vi "Periodic Tasks.vi"(8 "error in":errorcluster) -> ()   [LabVIEW 2023]
doc: "This VI runs in parallel to other robot code. It can contain as many user-defined periodic loops as you need. These can carry out PID or other sorts of timed response."
uses:
  MHZLib/Variables and Definitions/DB Auton Data.ctl
  <vilib>/Rock Robotics/WPI/ThirdParty/REV Robotics/REVLib/Typedef/Spark MAX Control Type.ctl
  <vilib>/Analysis/coordinate.llb/Angle Range (Degree).ctl
  <vilib>/Analysis/coordinate.llb/Angle Units.ctl
  MHZLib/Variables and Definitions/Auto_Values.ctl
  <vilib>/Rock Robotics/WPI/ThirdParty/Phoenix-LabVIEW/Pigeon IMU/CTRE_PigeonIMU_TareType.ctl
  c1e43d3c-3167-4efa-a61c-2a6e94be98fe.vi
  fdb43fbb-35d8-47d4-8d64-3b5a3af586d8.vi
  8a72de37-8128-41b9-abfb-9e0f917d53f3.vi
  <vilib>/Analysis/coordinate.llb/Wrap Angle (array).vi
  MHZLib/Variables and Definitions/Robot Global Data.vi
  <vilib>/Rock Robotics/Network Tables/NT Read Boolean.vi
  <vilib>/Rock Robotics/Network Tables/NT Read Float.vi
  <vilib>/addons/control/pid/pid.llb/PID (DBL).vi
  <vilib>/Rock Robotics/Network Tables/NT Write Number.vi
  <vilib>/Analysis/coordinate.llb/Angle Rotation (array).vi
  <vilib>/Analysis/coordinate.llb/Wrap Angle (scalar).vi
  <vilib>/Rock Robotics/WPI/ThirdParty/Phoenix-LabVIEW/Pigeon IMU/CTRE_PigeonIMU_GetYPR.vi
  <vilib>/Analysis/coordinate.llb/2D Cartesian Coordinate Rotation (Scalar).vi
  <vilib>/Rock Robotics/Network Tables/NT Read Numeric Array.vi
  <vilib>/Analysis/NI_AAL_Angle.lvlib
  <vilib>/Analysis/NI_AALPro.lvlib
  <vilib>/addons/control/pid/NI_PID_pid.lvlib
panel:
  in  "Speaker Pos":dbl
  in  "Amp Pos":dbl
  in  "Travel Pos":dbl
  in  "Intake Buffer":i16
  in  "Deliver Throttle":dbl
  in  "Intake Throttle":dbl
  out "Current Location":T1 {"Shooter Throttle" min=-360.0 max=360.0}
  in  "Strafe Tolerance":dbl
  in  "Rotate Tolerance":dbl
  in  "Target Rot":dbl
  in  "Target Y":dbl
  in  "Target X":dbl
  in  "Cancel":bool
  in  "Go To":bool
  in  "PID x":T2={"proportional gain (Kc)"=1.0, "integral time (Ti, min)"=0.01, "derivative time (Td, min)"=0.0} {"derivative time (Td, min)" format="%.3f"; "integral time (Ti, min)" format="%.3f"; "proportional gain (Kc)" format="%.3f"}
  in  "PID y":T2={"proportional gain (Kc)"=1.0, "integral time (Ti, min)"=0.01, "derivative time (Td, min)"=0.0} {"derivative time (Td, min)" format="%.3f"; "integral time (Ti, min)" format="%.3f"; "proportional gain (Kc)" format="%.3f"}
  in  "PID rot":T2={"proportional gain (Kc)"=1.0, "integral time (Ti, min)"=0.01, "derivative time (Td, min)"=0.0} {"derivative time (Td, min)" format="%.3f"; "integral time (Ti, min)" format="%.3f"; "proportional gain (Kc)" format="%.3f"}
  in  "Pod Offset":dbl[](array[numeric])=[90.0, 180.0, -90.0, 0.0]
  in  "Drive Mode":bool=TRUE caption="Gyro"
  in  "Reinit Gyro":bool
  out "BR Position":dbl
  out "FR Position":dbl
  out "BL Position":dbl
  out "FL Position":dbl
  out "Right X":dbl
  out "Left Y":dbl
  out "Left X":dbl
  in  "Drive Throttle":dbl
  in  "Drive dband":dbl
  in  "Steer dband":dbl
  out "FL Drive":dbl
  out "BL Drive":dbl
  out "FR Drive":dbl
  out "BR Drive":dbl
  out "Yaw":dbl
  in  "BR Steer":dbl
  in  "FR Steer":dbl
  in  "BL Steer":dbl
  in  "FL Steer":dbl
  # "I should probably look into why attempting to remove\nthis \"error in\" var completely breaks PT... or better yet,\nI should learn to implement proper error handling."
  # "This is some manual setpoint stuff for testing purposes"
  # "FL\n\nFR\n\nBR\n\nBL"
  # "ALWAYS have a backup plan!"
  # "Takes precedence\nfrom Tol"
  # "Relative"
  # "Absolute"
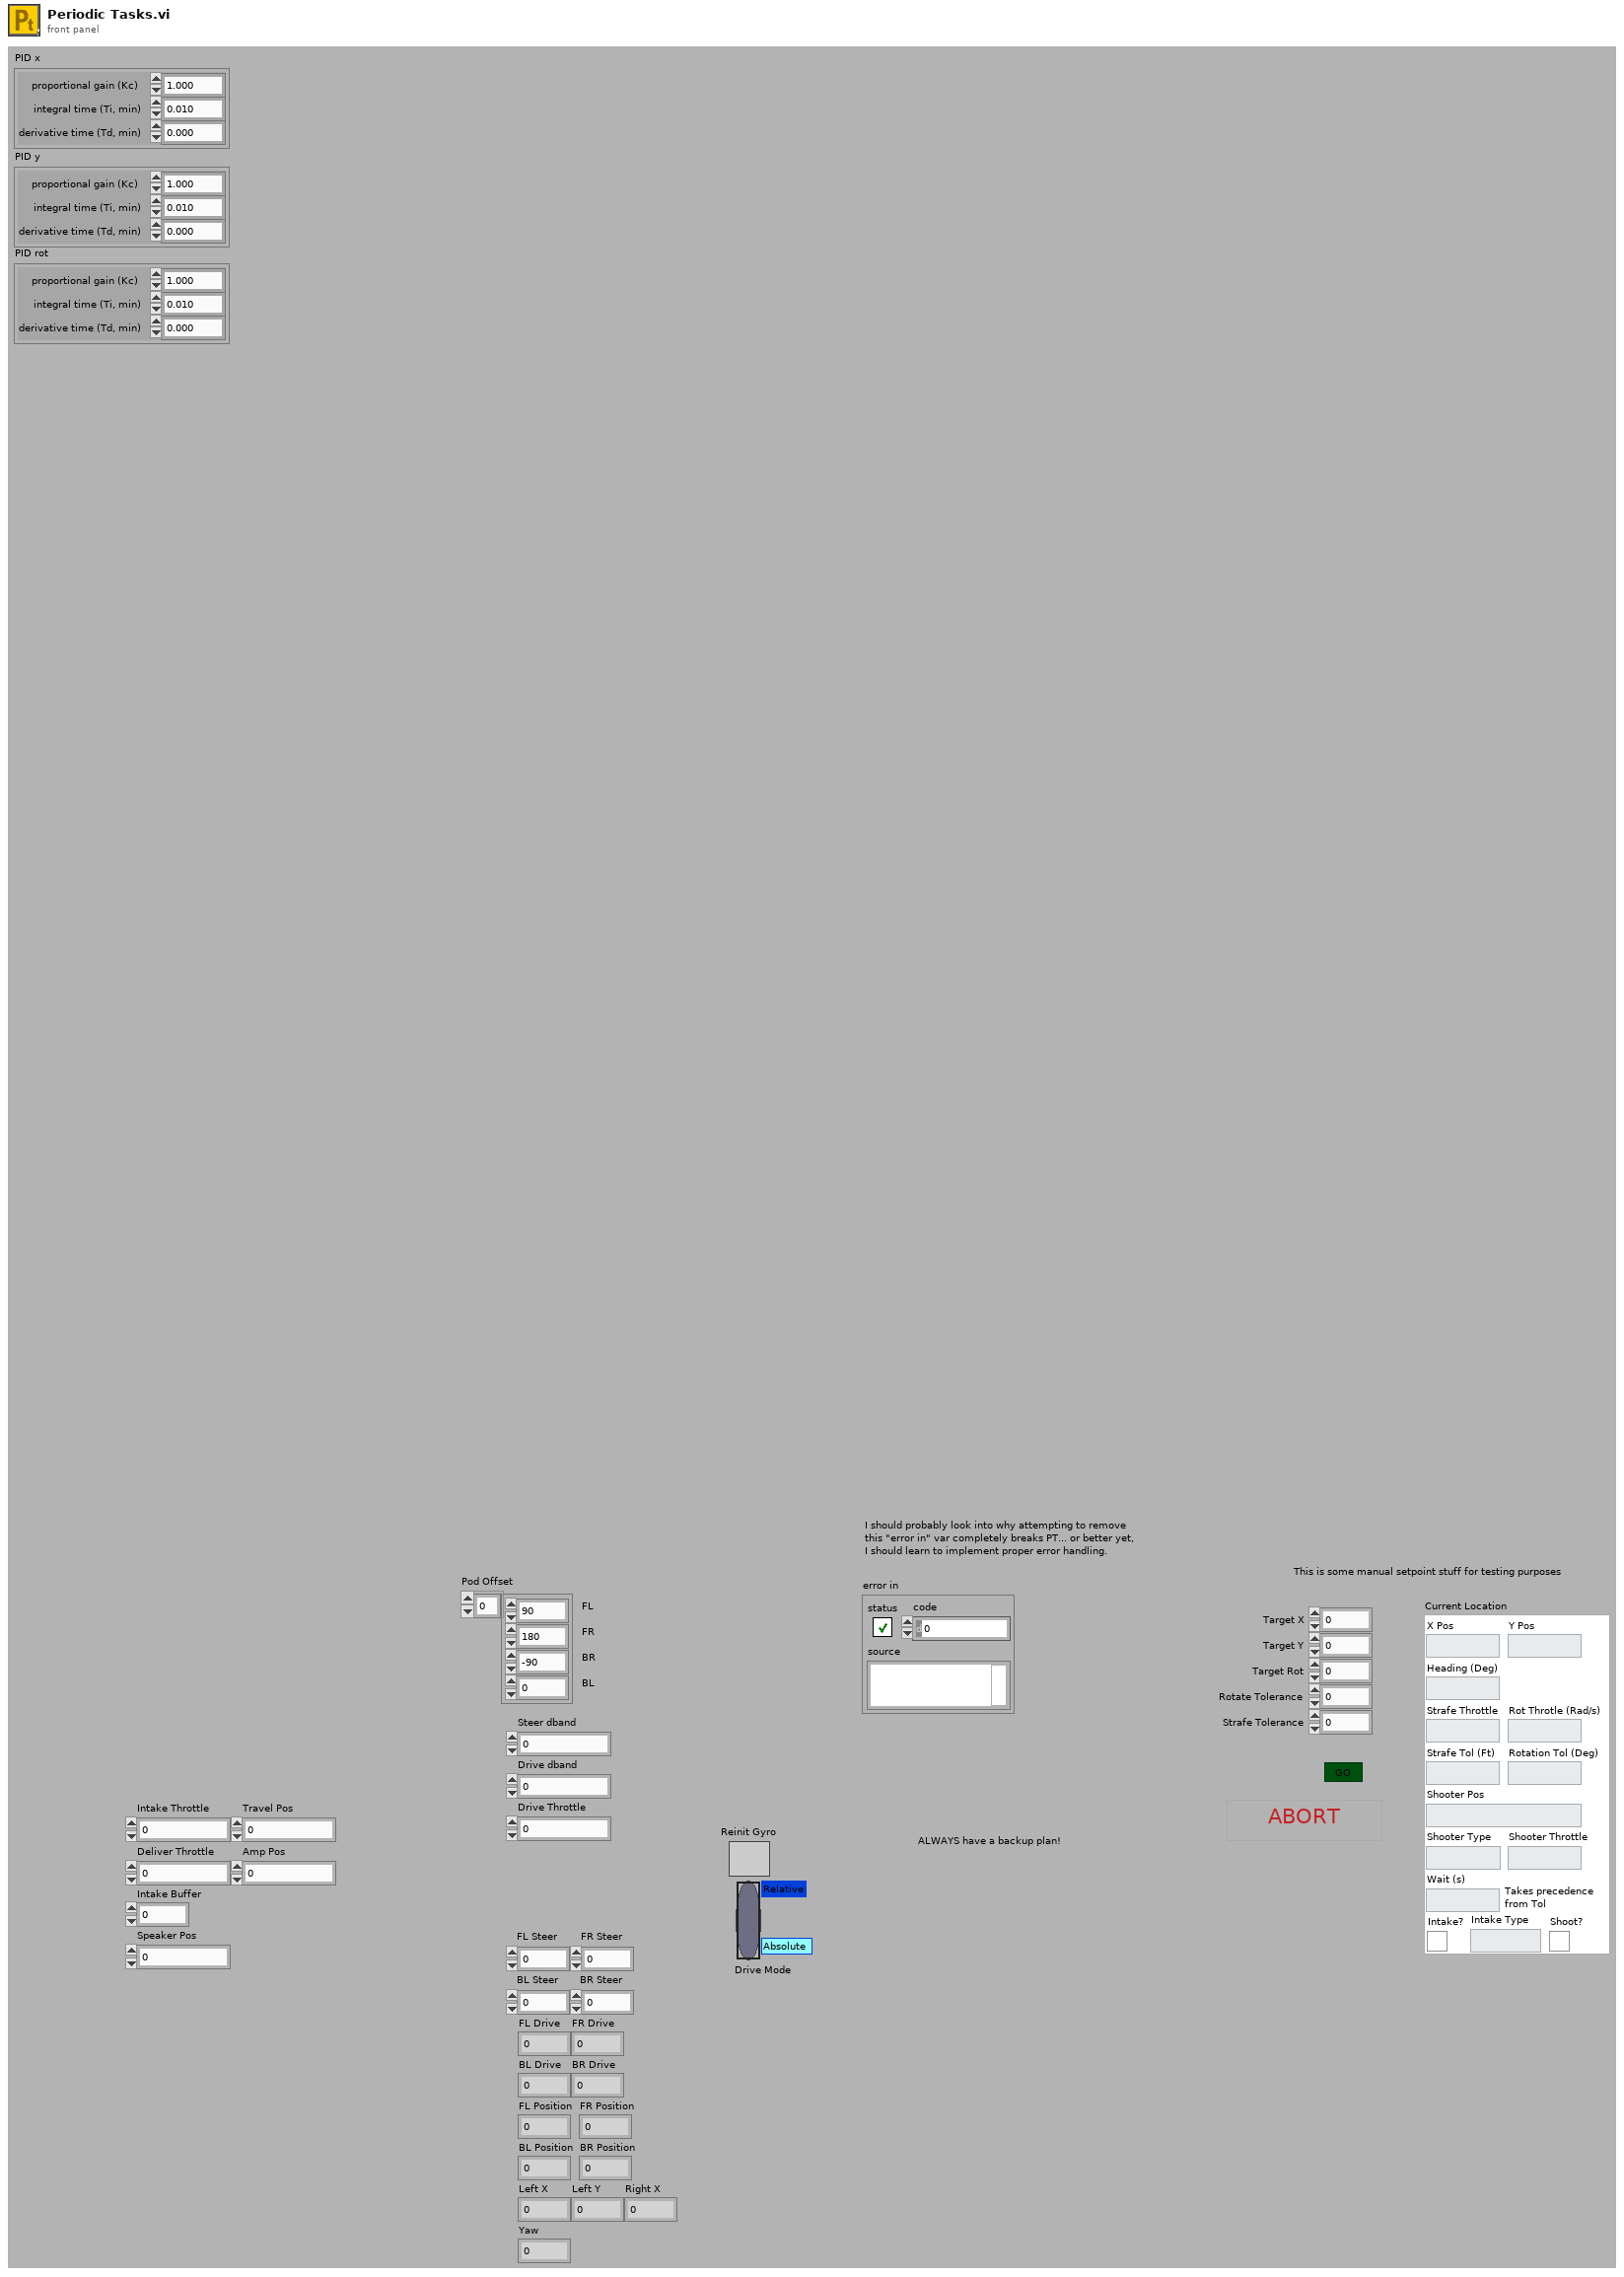
[diagram p1: front panel]
types:
  T1 = typedef "DB Auton Data.ctl" = cluster{"X Pos":dbl, "Y Pos":dbl, "Heading (Deg)":dbl, "Strafe Throttle":dbl, "Rot Throtle (Rad/s)":dbl, "Strafe Tol (Ft)":dbl, "Rotation Tol (Deg)":dbl, "Shooter Pos":enum16{"Travel", "Speaker", "Amp"}, "Intake Type":enum16{"Front", "Center"}, "Intake?":bool, "Shooter Type":enum16{"Manual", "Automatic"}, "Shooter Throttle":dbl, "Wait (s)":dbl, "Shoot?":bool}
  T2 = cluster{"proportional gain (Kc)":dbl, "integral time (Ti, min)":dbl, "derivative time (Td, min)":dbl}
  T3 = typedef "WPI_MotorControlDeviceRef.ctl" = cluster{"DeviceStatus":errorcluster, "Type":T4, "PWM":cluster{"PWM Channel":T5, "DeadBand":T6}, "CAN":cluster{"Device Number":u8, "SetOutput VI Ref":variant, "GetOutput VI Ref":variant, "Enable VI Ref":variant, "Disable VI Ref":variant, "Data":variant}, "Invert":bool, "DIO PWM":cluster{"PWM \"Enable\" Channel":T5, "DIOChannel":T7, "PWM Rate":dbl}}
  T4 = typedef "WPI_MotorControlType.ctl" = enum16{"PWM", "CAN", "DIO PWM"}
  T5 = typedef "FPGA_DIOPWMChannel.ctl" = enum8{"PWM 0", "PWM 1", "PWM 2", "PWM 3", "PWM 4", "PWM 5", "PWM 6", "PWM 7", "PWM 8", "PWM 9", "PWM MXP 0", "PWM MXP 1", "PWM MXP 2", "PWM MXP 3", "PWM MXP 4", "PWM MXP 5", "PWM MXP 6", "PWM MXP 7", "PWM MXP 8", "PWM MXP 9", "Invalid"}
  T6 = typedef "WPI_PWMDeadband.ctl" = cluster{"Name":string, "maxPositivePwm":i32, "minPositivePwm":i32, "centerPwm":i32, "maxNegativePwm":i32, "minNegativePwm":i32, "angularRange":u16}
  T7 = typedef "FPGA_DIOChannel.ctl" = enum8{"DIO 0", "DIO 1", "DIO 2", "DIO 3", "DIO 4", "DIO 5", "DIO 6", "DIO 7", "DIO 8", "DIO 9", "DIO MXP 0", "DIO MXP 1", "DIO MXP 2", "DIO MXP 3", "DIO MXP 4", "DIO MXP 5", "DIO MXP 6", "DIO MXP 7", "DIO MXP 8", "DIO MXP 9", "DIO MXP 10", "DIO MXP 11", "DIO MXP 12", "DIO MXP 13", "DIO MXP 14", "DIO MXP 15", "SPI Port CS1", "SPI Port CS2", "SPI Port CS3", "SPI Port MISO", "SPI Port MOSI", "Invalid"}
  T8 = typedef "Auto_Values.ctl" = cluster{"X Pos":dbl, "Y Pos":dbl, "Heading (Deg)":dbl, "Strafe Throttle":dbl, "Rot Throtle (Rad/s)":dbl, "Strafe Tol (Ft)":dbl, "Rotation Tol (Deg)":dbl, "Shooter Pos":enum16{"Travel", "Speaker", "Amp"}, "Intake Type":enum16{"Front", "Center"}, "Intake?":bool, "Shooter Type":enum16{"Manual", "Automatic"}, "Shooter Throttle":dbl, "Wait (s)":dbl, "Shoot?":bool}
  T9 = cluster{"value[0]":dbl, "value[1]":dbl, "value[2]":dbl, "value[3]":dbl, "value[4]":dbl, "value[5]":dbl, "value[6]":dbl, "value[7]":dbl, "value[8]":dbl}
  T10 = cluster{"Front Left":dbl[], "Front Right":dbl[], "Back Right":dbl[], "Back Left":dbl[]}
  T11 = typedef "NI_AAL_Angle.lvlib/Angle Units.ctl" = i32
  T12 = typedef "NI_AAL_Angle.lvlib/Angle Range (Degree).ctl" = u16
  T13 = typedef "CTRE_PigeonIMU_DeviceRef.ctl" = cluster{"DeviceStatus":errorcluster, "Device Number":u8, "Type":T14, "Device ID":u32, "Handle":u64, "UsageFrame":u32, "Library Path":path}
  T14 = typedef "CTRE_PigeonIMU_ConnectionType.ctl" = u32
  T15 = typedef "CTRE_PigeonIMU_TareType.ctl" = u8
  T16 = cluster{"FL Angle (rad)":dbl, "FL Velocity (ft/s)":dbl, "FR Angle (rad)":dbl, "FR Velocity (ft/s)":dbl, "BR Angle (rad)":dbl, "BR Velocity (ft/s)":dbl, "BL Angle (rad)":dbl, "BL Velocity (ft/s)":dbl}
  T17 = typedef "Spark MAX Control Type.ctl" = enum16{"Percent VBus", "Voltage", "Velocity", "Position", "Smart Motion", "Current", "Smart Velocity"}
  T18 = typedef "WPI_DigitalInputDevRef.ctl" = cluster{"DevStatus":errorcluster, "DIO Channel":T7}
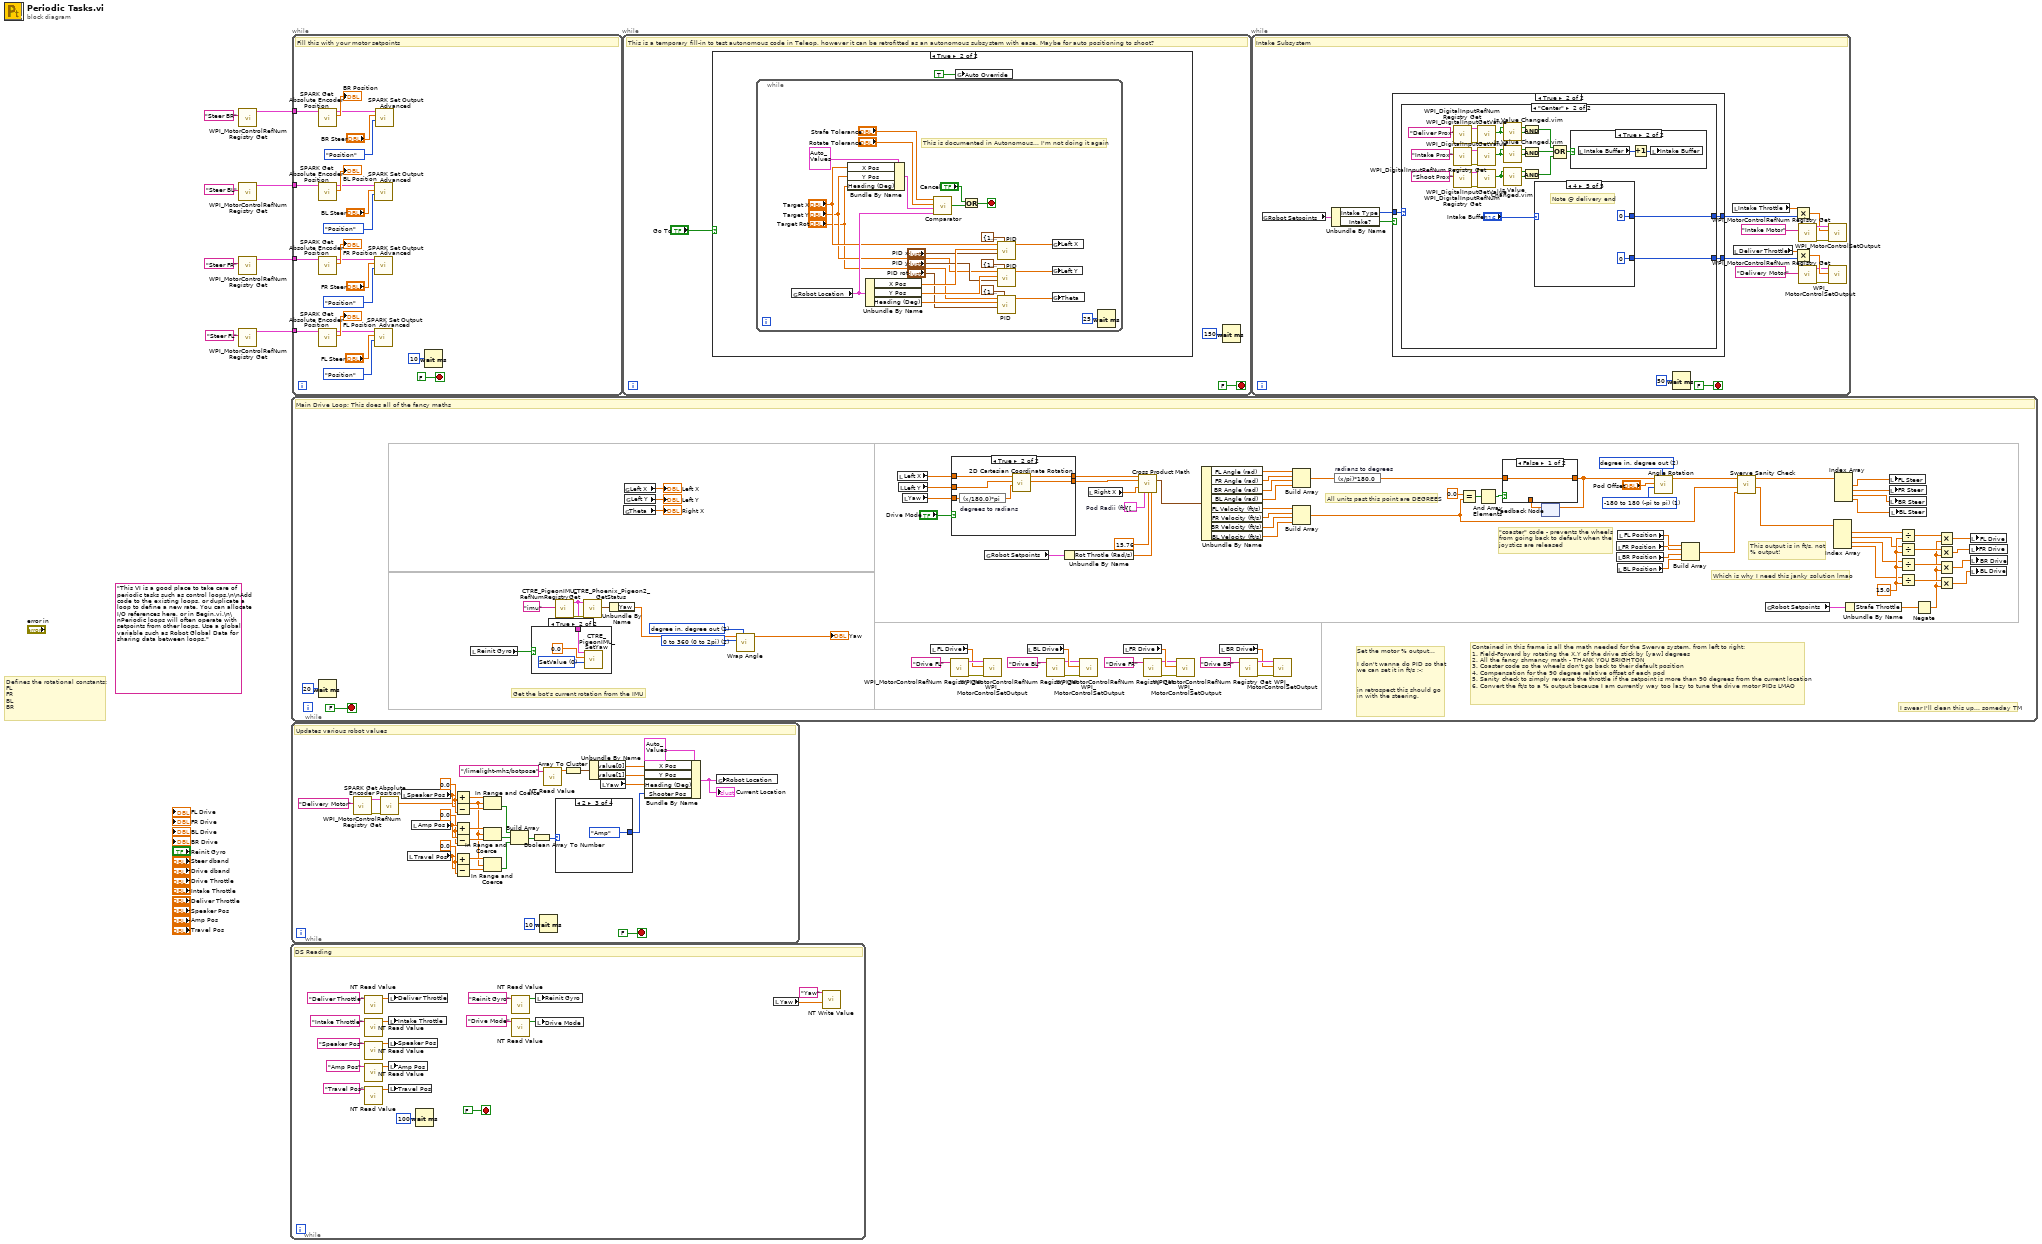
[diagram p0: block diagram]
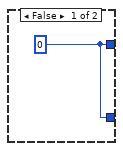
[diagram p2: hidden frame]
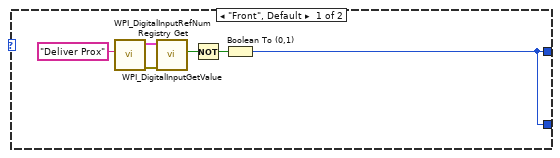
[diagram p3: hidden frame]
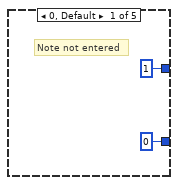
[diagram p5: hidden frame]
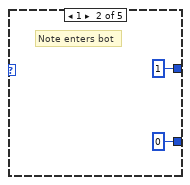
[diagram p6: hidden frame]
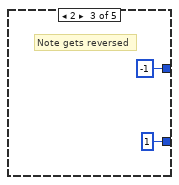
[diagram p7: hidden frame]
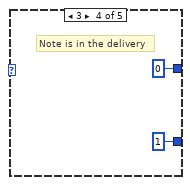
[diagram p8: hidden frame]
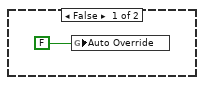
[diagram p9: hidden frame]
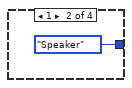
[diagram p11: hidden frame]
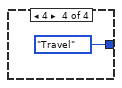
[diagram p12: hidden frame]
diagram:
  (unwired) "This VI is a good place to take care of periodic tasks such as control loops.\n\nAdd code to the existing loops, or duplicate a loop to define a new rate. You can allocate I/O references here, or in Begin.vi.\n\nPeriodic loops will often operate with setpoints from other loops. Use a global variable such as Robot Global Data for sharing data between loops."
  # "Defines the rotational constants:\nFL\nFR\nBL\nBR"
  n1 = call <vilib>:"WPI_MotorControlRefNum Registry Get.vi"("refnum name"="Steer BR" ("Change to match from begin.vi")) -> ("MotorControlDevRef"=w6:T3)  [unwired: 9 in, 1 out]
  n2 = call <vilib>:"WPI_MotorControlRefNum Registry Get.vi"("refnum name"="Steer BL" ("Change to match from begin.vi")) -> ("MotorControlDevRef"=w7:T3)  [unwired: 9 in, 1 out]
  n3 = call <vilib>:"WPI_MotorControlRefNum Registry Get.vi"("refnum name"="Steer FR" ("Change to match from begin.vi")) -> ("MotorControlDevRef"=w8:T3)  [unwired: 9 in, 1 out]
  n4 = call <vilib>:"WPI_MotorControlRefNum Registry Get.vi"("refnum name"="Steer FL" ("Change to match from begin.vi")) -> ("MotorControlDevRef"=w4:T3)  [unwired: 9 in, 1 out]
  n5 = while {
    stop <- FALSE stop-if-true
    # "DS Reading"
    n6 = call-poly <vilib>:"NT Read Value.vi"("name"="Deliver Throttle") -> ("value"=w15:dbl)  [unwired: 8 in, 2 out]
    n7 = call-poly <vilib>:"NT Read Value.vi"("name"="Intake Throttle") -> ("value"=w18:dbl)  [unwired: 8 in, 2 out]
    n8 = call-poly <vilib>:"NT Read Value.vi"("name"="Speaker Pos") -> ("value"=w14:dbl)  [unwired: 8 in, 2 out]
    n9 = call-poly <vilib>:"NT Read Value.vi"("name"="Amp Pos") -> ("value"=w11:dbl)  [unwired: 8 in, 2 out]
    n10 = call-poly <vilib>:"NT Read Value.vi"("name"="Travel Pos") -> ("value"=w10:dbl)  [unwired: 8 in, 2 out]
    n11 = local write "Deliver Throttle"(w15) -> ()
    n12 = local write "Intake Throttle"(w18) -> ()
    n13 = local write "Speaker Pos"(w14) -> ()
    n14 = local write "Amp Pos"(w11) -> ()
    n15 = local write "Travel Pos"(w10) -> ()
    n16 = Wait (ms)(milliseconds to wait=u32 100) -> ()  [unwired: 1 out]
    n17 = call-poly <vilib>:"NT Read Value.vi"("name"="Reinit Gyro") -> ("value"=w23:bool)  [unwired: 8 in, 2 out]
    n18 = call-poly <vilib>:"NT Read Value.vi"("name"="Drive Mode") -> ("value"=w22:bool)  [unwired: 8 in, 2 out]
    n19 = local write "Reinit Gyro"(w23) -> ()
    n20 = local write "Drive Mode"(w22) -> ()
    n21 = local read "Yaw"() -> (w19:dbl)
    n22 = call-poly <vilib>:"NT Write Value.vi"("value"=w19, "name"="Yaw") -> ()  [unwired: 9 in, 1 out]
  }
  n23 = while {
    stop <- FALSE stop-if-true
    w37 = 0.0 ("upper limit")
    w38 = 0.0 ("upper limit")
    w45 = 0.0 ("upper limit")
    # "Updates various robot values"
    n24 = call <vilib>:"WPI_MotorControlRefNum Registry Get.vi"("refnum name"="Delivery Motor" ("Change to match from begin.vi")) -> ("error out"=w47:errorcluster, "MotorControlDevRef"=w46:T3)  [unwired: 9 in]
    n25 = call <vilib>:"SPARK Get Absolute Encoder Position.vi"("error in (no error)"=w47, "MotorControlDeviceRef in"=w46) -> ("Position"=w33:dbl)  [unwired: 6 in, 3 out]
    n26 = local read "Speaker Pos"() -> (w44:dbl)
    n27 = local read "Travel Pos"() -> (w36:dbl)
    n28 = local read "Amp Pos"() -> (w39:dbl)
    n29 = Add(x=w44, y=w45) -> (x+y=w42:dbl)
    n30 = Subtract(x=w44, y=w45) -> (x-y=w43:dbl)
    n31 = Add(x=w39, y=w38) -> (x+y=w41:dbl)
    n32 = Subtract(x=w39, y=w38) -> (x-y=w40:dbl)
    n33 = Add(x=w36, y=w37) -> (x+y=w34:dbl)
    n34 = Subtract(x=w36, y=w37) -> (x-y=w35:dbl)
    n35 = In Range and Coerce(upper limit=w42, x=w33, lower limit=w43) -> (In Range?=w31:bool)  [unwired: 1 out]
    n36 = In Range and Coerce(upper limit=w41, x=w33, lower limit=w40) -> (In Range?=w32:bool)  [unwired: 1 out]
    n37 = In Range and Coerce(upper limit=w34, x=w33, lower limit=w35) -> (In Range?=w30:bool)  [unwired: 1 out]
    n38 = Build Array(w31, w32, w30) -> (w29:bool[])
    n39 = Boolean Array To Number(Boolean array=w29) -> (number=w28:u32)
    n40 = Wait (ms)(milliseconds to wait=u32 10) -> ()  [unwired: 1 out]
    n41 = call-poly <vilib>:"NT Read Value.vi"("name"="/limelight-mhz/botpose" ("Name")) -> ("value"=w54:dbl[])  [unwired: 8 in, 2 out]
    n42 = case shown="2" w28 {
      tunnel: [_ enum16{"Travel", "Speaker", "Amp"}."Speaker" ("Shooter Pos") enum16{"Travel", "Speaker", "Amp"}."Amp" ("Shooter Pos") enum16{"Travel", "Speaker", "Amp"}."Travel" ("Shooter Pos")] -> w27
      frame 0, Default {
      }
      frame 1 {
      }
      frame 2 {
      }
      frame 4 {
      }
    }
    n43 = Array To Cluster(array=w54) -> (cluster=w53:T9)
    n44 = Unbundle By Name(w53) -> ("value[0]"=w52:dbl, "value[1]"=w51:dbl)
    n45 = local read "Yaw"() -> (w57:dbl)
    n46 = Bundle By Name(cluster=T8 {"X Pos"=0.0, "Y Pos"=0.0, "Heading (Deg)"=0.0, "Strafe Throttle"=0.0, "Rot Throtle (Rad/s)"=0.0, "Strafe Tol (Ft)"=0.0, "Rotation Tol (Deg)"=0.0, "Shooter Pos"=enum."Travel", "Intake Type"=enum."Front", "Intake?"=FALSE, "Shooter Type"=enum."Manual", "Shooter Throttle"=0.0, "Wait (s)"=0.0, "Shoot?"=FALSE} ("element"), "X Pos"=w52, "Y Pos"=w51, "Heading (Deg)"=w57, "Shooter Pos"=w27) -> (w49:T8)
    "Current Location" <- w49
    n47 = global write "Robot Global Data.vi" "Robot Location"(w49) -> ()
  }
  n48 = while {
    stop <- FALSE stop-if-true
    w77 = T10 {"Front Left"=[11.0, 11.0, 0.0], "Front Right"=[-11.0, 11.0, 0.0], "Back Right"=[-11.0, -11.0, 0.0], "Back Left"=[11.0, -11.0, 0.0]}  # Pod Radii (ft)
    w100 = T11 2 items=["radian in, radian out", "radian in, degree out", "degree in, degree out", "degree in, radian out"] ("angle units")
    w101 = T12 2 items=["none", "-180 to 180 (-pi to pi)", "0 to 360 (0 to 2pi)"] ("angle range")
    w128 = T11 2 items=["radian in, radian out", "radian in, degree out", "degree in, degree out", "degree in, radian out"] ("angle units")
    w129 = T12 1 items=["none", "-180 to 180 (-pi to pi)", "0 to 360 (0 to 2pi)"] ("rotated angle range")
    w130 = 15.0 ("y")
    # "Which is why I need this janky solution lmao"
    # "Set the motor % output...\n\nI don't wanna do PID so that\nwe can set it in ft/s ;-;\n\n\nin retrospect this should go\nin with the steering."
    # "This output is in ft/s, not\n% output!"
    # "Contained in this frame is all the math needed for the Swerve system, from left to right:\n1. Field-Forward by rotating the X,Y of the drive stick by [yaw] degrees\n2. All the fancy shmancy math - THANK YOU BRIGHTON\n3. Coaster code so the wheels don't go back to their default position\n4. Compensation for the 90 degree relative offset of each pod\n5. Sanity check to simply reverse the throttle if the setpoint is more than 90 degrees from the current location\n6. Convert the ft/s to a % output because I am currently way too lazy to tune the drive motor PIDs LMAO"
    # "\"coaster\" code - prevents the wheels\nfrom going back to default when the\njoystics are released"
    # "I swear I'll clean this up... someday TM"
    # "All units past this point are DEGREES"
    # "Get the bot's current rotation from the IMU"
    # "Main Drive Loop; This does all of the fancy maths"
    n49 = Wait (ms)(milliseconds to wait=u32 20) -> ()  [unwired: 1 out]
    n50 = local read "Reinit Gyro"() -> (w70:bool)
    n51 = call <vilib>:"CTRE_PigeonIMU_RefNumRegistryGet.vi"("refnum name"="imu") -> ("error out"=w73:errorcluster, "PigeonIMUDevRef"=w71:T13)  [unwired: 9 in]
    n52 = case shown="True" w70 {
      tunnel: w71 -> [_ w153]
      frame False {
      }
      frame True {
        w152 = T15 0 items=["SetValue"=0, "AddOffset"=1, "MatchCompass"=2, "SetOffset"=255] ("TareType (SetValue)")
        n53 = call <vilib>:"CTRE_PigeonIMU_SetYaw.vi"("TareType (SetValue)"=w152, "Value"=0.0, "PigeonIMUDevRef"=w153) -> ()  [unwired: 7 in, 2 out]
      }
    }
    n54 = call-poly <vilib>:"CTRE_Phoenix_Pigeon2_GetStatus.vi"("error in (no error)"=w73, "PigeonIMUDevRef"=w71) -> ("Yaw Pitch Roll"=w69:cluster{"Yaw":dbl, "Pitch":dbl, "Roll":dbl})  [unwired: 7 in, 2 out]
    n55 = Unbundle By Name(w69) -> ("Yaw"=w88:dbl)
    n56 = global read "Robot Global Data.vi" "Theta"() -> (→"Right X":dbl)
    n57 = global read "Robot Global Data.vi" "Left X"() -> (→"Left X":dbl)
    n58 = global read "Robot Global Data.vi" "Left Y"() -> (→"Left Y":dbl)
    n59 = call-poly <vilib>:"Wrap Angle.vi"("angle units"=w100, "angle range"=w101, "angle in"=w88) -> ("angle out"=→"Yaw":dbl)  [unwired: 7 in, 1 out]
    n60 = local read "Left X"() -> (w94:dbl)
    n61 = local read "Left Y"() -> (w93:dbl)
    n62 = local read "Yaw"() -> (w89:dbl)
    n63 = local read "FL Drive"() -> (w145:dbl)
    n64 = call <vilib>:"WPI_MotorControlRefNum Registry Get.vi"("refnum name"="Drive FL") -> ("error out"=w147:errorcluster, "MotorControlDevRef"=w146:T3)  [unwired: 9 in]
    n65 = case shown="True" "Drive Mode" {
      tunnel: w94 -> [w155 w160]
      tunnel: w93 -> [w154 w161]
      tunnel: [w155 w159] -> w91
      tunnel: [w154 w158] -> w90
      tunnel: w89 -> [_ w156]
      frame False {
      }
      frame True {
        n66 = expression code="(x/180.0)*pi" "degrees to radians"(w156) -> (w157:dbl)
        n67 = call-poly <vilib>:"2D Cartesian Coordinate Rotation.vi"("theta"=w157, "y"=w161, "x"=w160) -> ("y out"=w158:dbl, "x out"=w159:dbl)  [unwired: 6 in, 1 out]
      }
    }
    n68 = call <vilib>:"WPI_MotorControlSetOutput.vi"("error in (no error)"=w147, "Output"=w145, "MotorControlDevRef"=w146) -> ()  [unwired: 6 in, 3 out]
    n69 = global read "Robot Global Data.vi" "Robot Setpoints"() -> (w74:T8)
    n70 = local read "BL Drive"() -> (w144:dbl)
    n71 = call <vilib>:"WPI_MotorControlRefNum Registry Get.vi"("refnum name"="Drive BL") -> ("error out"=w142:errorcluster, "MotorControlDevRef"=w143:T3)  [unwired: 9 in]
    n72 = Unbundle By Name(w74) -> ("Rot Throtle (Rad/s)"=w68:dbl)
    n73 = call <vilib>:"WPI_MotorControlSetOutput.vi"("error in (no error)"=w142, "Output"=w144, "MotorControlDevRef"=w143) -> ()  [unwired: 6 in, 3 out]
    n74 = local read "Right X"() -> (w132:dbl)
    n75 = local read "FR Drive"() -> (w136:dbl)
    n76 = call "Cross Product Math.vi"("Left X"=w91, "Left Y"=w90, "Right X"=w132, "Radii (ft)"=w77, "Max Speed (ft/s)"=15.76, "Max Rotation (rad/s)"=w68) -> ("Modules Out"=w131:T16)  [unwired: 9 in]
    n77 = call <vilib>:"WPI_MotorControlRefNum Registry Get.vi"("refnum name"="Drive FR") -> ("error out"=w134:errorcluster, "MotorControlDevRef"=w135:T3)  [unwired: 9 in]
    n78 = call <vilib>:"WPI_MotorControlSetOutput.vi"("error in (no error)"=w134, "Output"=w136, "MotorControlDevRef"=w135) -> ()  [unwired: 6 in, 3 out]
    n79 = Unbundle By Name(w131) -> ("FL Angle (rad)"=w126:dbl, "FR Angle (rad)"=w125:dbl, "BR Angle (rad)"=w124:dbl, "BL Angle (rad)"=w123:dbl, "FL Velocity (ft/s)"=w109:dbl, "FR Velocity (ft/s)"=w108:dbl, "BR Velocity (ft/s)"=w107:dbl, "BL Velocity (ft/s)"=w106:dbl)
    n80 = local read "BR Drive"() -> (w137:dbl)
    n81 = call <vilib>:"WPI_MotorControlRefNum Registry Get.vi"("refnum name"="Drive BR") -> ("error out"=w139:errorcluster, "MotorControlDevRef"=w138:T3)  [unwired: 9 in]
    n82 = call <vilib>:"WPI_MotorControlSetOutput.vi"("error in (no error)"=w139, "Output"=w137, "MotorControlDevRef"=w138) -> ()  [unwired: 6 in, 3 out]
    n83 = Build Array(w126, w125, w124, w123) -> (w67:dbl[])
    n84 = Build Array(w109, w108, w107, w106) -> (w66:dbl[])
    n85 = expression code="(x/pi)*180.0" "radians to degrees"(w67) -> (w83:dbl[])
    n86 = Equal?(x=0.0, y=w66) -> (x = y?=w98:bool[])
    n87 = And Array Elements(Boolean array=w98) -> (logical AND=w97:bool)
    n88 = feedback #1() -> (w95:dbl[])  [unwired: 1 in]
    n89 = case shown="False" w97 {
      tunnel: [w162 w163] -> w96
      tunnel: w83 -> [w162 _]
      tunnel: w95 -> [_ w163]
      frame False {
      }
      frame True {
      }
    }
    n90 = feedback-in #1(w96) -> ()
    n91 = local read "FR Position"() -> (w84:dbl)
    n92 = local read "BR Position"() -> (w85:dbl)
    n93 = local read "BL Position"() -> (w86:dbl)
    n94 = local read "FL Position"() -> (w87:dbl)
    n95 = call-poly <vilib>:"Angle Rotation.vi"("angle units"=w128, "rotated angle range"=w129, "Counterclockwise Rotation"="Pod Offset", "Angle"=w96) -> ("Rotated Angle"=w82:dbl[])  [unwired: 6 in, 1 out]
    n96 = Build Array(w87, w84, w85, w86) -> (w79:dbl[])
    n97 = call "Swerve Sanity Check.vi"("Current Pod Setpoints"=w79, "Throttle In"=w66, "Steer In"=w82) -> ("Throttle Out"=w80:dbl[], "Steer Out"=w81:dbl[])  [unwired: 3 in]
    n98 = global read "Robot Global Data.vi" "Robot Setpoints"() -> (w75:T8)
    n99 = Index Array(array=w80) -> (element #1=w105:dbl, element #2=w104:dbl, element #3=w103:dbl, element #4=w102:dbl)  [unwired: 4 in]
    n100 = Index Array(array=w81) -> (element #1=w122:dbl, element #2=w121:dbl, element #3=w120:dbl, element #4=w119:dbl)  [unwired: 4 in]
    n101 = Unbundle By Name(w75) -> ("Strafe Throttle"=w65:dbl)
    n102 = local write "FL Steer"(w122) -> ()
    n103 = local write "FR Steer"(w121) -> ()
    n104 = local write "BR Steer"(w120) -> ()
    n105 = local write "BL Steer"(w119) -> ()
    n106 = Divide(x=w105, y=w130) -> (x/y=w115:dbl)
    n107 = Divide(x=w104, y=w130) -> (x/y=w116:dbl)
    n108 = Divide(x=w103, y=w130) -> (x/y=w117:dbl)
    n109 = Divide(x=w102, y=w130) -> (x/y=w118:dbl)
    n110 = Negate(x=w65) -> (-x=w110:dbl)
    n111 = Multiply(x=w115, y=w110) -> (x*y=w114:dbl)
    n112 = Multiply(x=w116, y=w110) -> (x*y=w113:dbl)
    n113 = Multiply(x=w117, y=w110) -> (x*y=w112:dbl)
    n114 = Multiply(x=w118, y=w110) -> (x*y=w111:dbl)
    n115 = local write "FR Drive"(w113) -> ()
    n116 = local write "FL Drive"(w114) -> ()
    n117 = local write "BR Drive"(w112) -> ()
    n118 = local write "BL Drive"(w111) -> ()
  }
  n119 = while {
    tunnel: w4 -> [w174]
    tunnel: w8 -> [w172]
    tunnel: w7 -> [w170]
    tunnel: w6 -> [w168]
    stop <- FALSE stop-if-true
    # "Fill this with your motor setpoints"
    n120 = call <vilib>:"SPARK Get Absolute Encoder Position.vi"("MotorControlDeviceRef in"=w168) -> ("Position"=→"BR Position":dbl, "MotorControlDeviceRef out"=w164:T3)  [unwired: 7 in, 2 out]
    n121 = call <vilib>:"SPARK Get Absolute Encoder Position.vi"("MotorControlDeviceRef in"=w170) -> ("Position"=→"BL Position":dbl, "MotorControlDeviceRef out"=w165:T3)  [unwired: 7 in, 2 out]
    n122 = call <vilib>:"SPARK Get Absolute Encoder Position.vi"("MotorControlDeviceRef in"=w172) -> ("Position"=→"FR Position":dbl, "MotorControlDeviceRef out"=w166:T3)  [unwired: 7 in, 2 out]
    n123 = call <vilib>:"SPARK Get Absolute Encoder Position.vi"("MotorControlDeviceRef in"=w174) -> ("Position"=→"FL Position":dbl, "MotorControlDeviceRef out"=w167:T3)  [unwired: 7 in, 2 out]
    n124 = call <vilib>:"SPARK Set Output Advanced.vi"("Control Mode"=Spark_MAX_Control_Type."Position", "Setpoint"="FL Steer", "MotorControlDevRef"=w167) -> ()  [unwired: 7 in, 2 out]
    n125 = call <vilib>:"SPARK Set Output Advanced.vi"("Control Mode"=Spark_MAX_Control_Type."Position", "Setpoint"="BL Steer", "MotorControlDevRef"=w165) -> ()  [unwired: 7 in, 2 out]
    n126 = call <vilib>:"SPARK Set Output Advanced.vi"("Control Mode"=Spark_MAX_Control_Type."Position", "Setpoint"="FR Steer", "MotorControlDevRef"=w166) -> ()  [unwired: 7 in, 2 out]
    n127 = call <vilib>:"SPARK Set Output Advanced.vi"("Control Mode"=Spark_MAX_Control_Type."Position", "Setpoint"="BR Steer", "MotorControlDevRef"=w164) -> ()  [unwired: 7 in, 2 out]
    n128 = Wait (ms)(milliseconds to wait=u32 10) -> ()  [unwired: 1 out]
  }
  n129 = while {
    stop <- FALSE stop-if-true
    # "This is a temporary fill-in to test autonomous code in Teleop, however it can be retrofitted as an autonomous subsystem with ease. Maybe for auto positioning to shoot?"
    n130 = case shown="True" "Go To" {
      frame False {
        n131 = global write "Robot Global Data.vi" "Auto Override"(FALSE ("Auto Override")) -> ()
      }
      frame True {
        n132 = while {
          stop <- w195 stop-if-true
          # "This is documented in Autonomous... I'm not doing it again"
          n133 = global read "Robot Global Data.vi" "Robot Location"() -> (w210:T8)
          n134 = Bundle By Name(cluster=T8 {"X Pos"=0.0, "Y Pos"=0.0, "Heading (Deg)"=0.0, "Strafe Throttle"=0.0, "Rot Throtle (Rad/s)"=0.0, "Strafe Tol (Ft)"=0.0, "Rotation Tol (Deg)"=0.0, "Shooter Pos"=enum."Travel", "Intake Type"=enum."Front", "Intake?"=FALSE, "Shooter Type"=enum."Manual", "Shooter Throttle"=0.0, "Wait (s)"=0.0, "Shoot?"=FALSE} ("element"), "X Pos"="Target X", "Y Pos"="Target Y", "Heading (Deg)"="Target Rot") -> (w198:T8)
          n135 = Unbundle By Name(w210) -> ("X Pos"=w209:dbl, "Y Pos"=w208:dbl, "Heading (Deg)"=w207:dbl)
          n136 = call "Comparator.vi"("Current Location"=w210, "Target Location"=w198, "Rotate Tolerance"="Rotate Tolerance", "Strafe Tolerance"="Strafe Tolerance") -> ("In range?"=w197:bool)
          n137 = Or(x="Cancel", y=w197) -> (x .or. y?=w195:bool)
          n138 = call-poly <vilib>:"PID.vi"("output range"=cluster{"output high":dbl, "output low":dbl} {"output high"=1.0, "output low"=-1.0}, "PID gains"="PID x", "process variable"=w209, "setpoint"="Target X") -> ("output"=w203:dbl)  [unwired: 6 in, 1 out]
          n139 = call-poly <vilib>:"PID.vi"("output range"=cluster{"output high":dbl, "output low":dbl} {"output high"=1.0, "output low"=-1.0}, "PID gains"="PID y", "process variable"=w208, "setpoint"="Target Y") -> ("output"=w191:dbl)  [unwired: 6 in, 1 out]
          n140 = call-poly <vilib>:"PID.vi"("output range"=cluster{"output high":dbl, "output low":dbl} {"output high"=1.0, "output low"=-1.0}, "PID gains"="PID rot", "process variable"=w207, "setpoint"="Target Rot") -> ("output"=w192:dbl)  [unwired: 6 in, 1 out]
          n141 = global write "Robot Global Data.vi" "Left X"(w203) -> ()
          n142 = global write "Robot Global Data.vi" "Left Y"(w191) -> ()
          n143 = global write "Robot Global Data.vi" "Theta"(w192) -> ()
          n144 = Wait (ms)(milliseconds to wait=u32 25) -> ()  [unwired: 1 out]
        }
        n145 = global write "Robot Global Data.vi" "Auto Override"(TRUE ("Auto Override")) -> ()
      }
    }
    n146 = Wait (ms)(milliseconds to wait=u32 150) -> ()  [unwired: 1 out]
  }
  n147 = while {
    stop <- FALSE stop-if-true
    # "Intake Subsystem"
    n148 = global read "Robot Global Data.vi" "Robot Setpoints"() -> (w229:T8)
    n149 = Unbundle By Name(w229) -> ("Intake Type"=w227:enum16{"Front", "Center"}, "Intake?"=w228:bool)
    n150 = case shown="True" w228 {
      tunnel: w227 -> [_ w235]
      tunnel: [w232 w234] -> w222
      tunnel: [w232 w233] -> w215
      frame False {
        w232 = i16 0 ("Intake Buffer")
      }
      frame True {
        n151 = case shown="\"Center\"" w235 {
          tunnel: [w236 w259] -> w234
          tunnel: [w236 w258] -> w233
          frame "Front", Default {
            n152 = call <vilib>:"WPI_DigitalInputRefNum Registry Get.vi"("refnum name"="Deliver Prox") -> ("error out"=w241:errorcluster, "DigitalInputDevRef"=w240:T18)  [unwired: 9 in]
            n153 = call <vilib>:"WPI_DigitalInputGetValue.vi"("error in (no error)"=w241, "DigitalInputDevRef"=w240) -> ("Value"=w239:bool)  [unwired: 7 in, 2 out]
            n154 = Not(x=w239) -> (.not. x?=w237:bool)
            n155 = Boolean To (0,1)(Boolean=w237) -> (0, 1=w236:i16)
          }
          frame "Center" {
            n156 = call <vilib>:"WPI_DigitalInputRefNum Registry Get.vi"("refnum name"="Deliver Prox") -> ("error out"=w252:errorcluster, "DigitalInputDevRef"=w253:T18)  [unwired: 9 in]
            n157 = call <vilib>:"WPI_DigitalInputRefNum Registry Get.vi"("refnum name"="Intake Prox") -> ("error out"=w263:errorcluster, "DigitalInputDevRef"=w262:T18)  [unwired: 9 in]
            n158 = call <vilib>:"WPI_DigitalInputRefNum Registry Get.vi"("refnum name"="Shoot Prox") -> ("error out"=w246:errorcluster, "DigitalInputDevRef"=w242:T18)  [unwired: 9 in]
            n159 = call <vilib>:"WPI_DigitalInputGetValue.vi"("error in (no error)"=w252, "DigitalInputDevRef"=w253) -> ("Value"=w243:bool)  [unwired: 7 in, 2 out]
            n160 = call <vilib>:"WPI_DigitalInputGetValue.vi"("error in (no error)"=w263, "DigitalInputDevRef"=w262) -> ("Value"=w256:bool)  [unwired: 7 in, 2 out]
            n161 = call <vilib>:"WPI_DigitalInputGetValue.vi"("error in (no error)"=w246, "DigitalInputDevRef"=w242) -> ("Value"=w244:bool)  [unwired: 7 in, 2 out]
            n162 = call "Is Value Changed.vim"("value"=w243) -> ("changed or first call?"=w255:bool)
            n163 = call "Is Value Changed.vim"("value"=w256) -> ("changed or first call?"=w257:bool)
            n164 = call "Is Value Changed.vim"("value"=w244) -> ("changed or first call?"=w248:bool)
            n165 = And(x=w243, y=w255) -> (x .and. y?=w250:bool)
            n166 = And(x=w256, y=w257) -> (x .and. y?=w249:bool)
            n167 = And(x=w244, y=w248) -> (x .and. y?=w245:bool)
            n168 = case shown="4" "Intake Buffer" {
              tunnel: [i16 1 ("Intake Buffer") i16 1 ("Intake Buffer") i16 -1 ("Intake Buffer") i16 0 ("Intake Buffer") i16 0 ("Intake Buffer")] -> w259
              tunnel: [i16 0 ("Intake Buffer") i16 0 ("Intake Buffer") i16 1 ("Intake Buffer") i16 1 ("Intake Buffer") i16 0 ("Intake Buffer")] -> w258
              frame 0, Default {
                # "Note not entered"
              }
              frame 1 {
                # "Note enters bot"
              }
              frame 2 {
                # "Note gets reversed"
              }
              frame 3 {
                # "Note is in the delivery"
              }
              frame 4 {
                # "Note @ delivery end"
              }
            }
            n169 = Compound Arithmetic op=OR(w250, w249, w245) -> (w251:bool)
            n170 = case shown="True" w251 {
              frame False {
              }
              frame True {
                n171 = local read "Intake Buffer"() -> (w265:i16)
                n172 = Increment(x=w265) -> (x+1=w264:i16)
                n173 = local write "Intake Buffer"(w264) -> ()
              }
            }
          }
        }
      }
    }
    n174 = Wait (ms)(milliseconds to wait=u32 50) -> ()  [unwired: 1 out]
    n175 = local read "Intake Throttle"() -> (w221:dbl)
    n176 = local read "Deliver Throttle"() -> (w220:dbl)
    n177 = Multiply(x=w221, y=w222) -> (x*y=w223:dbl)
    n178 = Multiply(x=w220, y=w215) -> (x*y=w219:dbl)
    n179 = call <vilib>:"WPI_MotorControlRefNum Registry Get.vi"("refnum name"="Intake Motor") -> ("error out"=w225:errorcluster, "MotorControlDevRef"=w226:T3)  [unwired: 9 in]
    n180 = call <vilib>:"WPI_MotorControlRefNum Registry Get.vi"("refnum name"="Delivery Motor") -> ("error out"=w218:errorcluster, "MotorControlDevRef"=w217:T3)  [unwired: 9 in]
    n181 = call <vilib>:"WPI_MotorControlSetOutput.vi"("error in (no error)"=w225, "Output"=w223, "MotorControlDevRef"=w226) -> ()  [unwired: 6 in, 3 out]
    n182 = call <vilib>:"WPI_MotorControlSetOutput.vi"("error in (no error)"=w218, "Output"=w219, "MotorControlDevRef"=w217) -> ()  [unwired: 6 in, 3 out]
  }
